vi "SV Read Next Measurement Data.vi"(5 "test signal configuration":refnum<class "SV Signal.lvclass">, 6 "reset start (F)":bool, 7 "reader ID":string="MeasurementData", 8 "error in (no error)":errorcluster, 9 "timeout (1000 ms)":i32=1000, 10 "block length (-1 = all)":i32=-1, 11 "buffer":refnum<data-value>) -> (0 "error out":errorcluster, 1 "end of buffer":bool, 2 "waveforms subset":waveform(dbl)[](array[waveform]), 3 "buffer out":refnum<data-value>, 4 "done":bool)   [LabVIEW 2017]
doc: "Adds buffering to stimulus-response applications. You must manually select the polymorphic instance to use."
uses:
  <vilib>/addons/_NISVFA/_Generation/Signal Generation/SV Signal/SV Signal.lvclass
  <vilib>/addons/_NISVFA/_Shared subVIs/Data Objects/Waveforms (DBL)/Waveforms (N Ch).lvclass
  C:/Program Files (x86)/National Instruments/LabVIEW 2017/vi.lib/addons/_NISVFA/_Shared subVIs/Data Objects/Data/Data.lvclass
  <vilib>/addons/_NISVFA/_Shared subVIs/Data Objects/Data/Data.lvclass/Data.ctl
  <vilib>/addons/_NISVFA/_Shared subVIs/Common/sv_Get NI Property Name String.vi
  <vilib>/addons/_NISVFA/_Generation/Signal Generation/SV Signal/Write Sample Rate.vi
  <vilib>/addons/_NISVFA/_Generation/Signal Generation/SV Signal/Read Sample Rate.vi
  <vilib>/addons/_NISVFA/_Shared subVIs/Data Objects/Data/Data.lvclass
  <vilib>/addons/_NISVFA/_Generation/SoundVib_Generation.lvlib
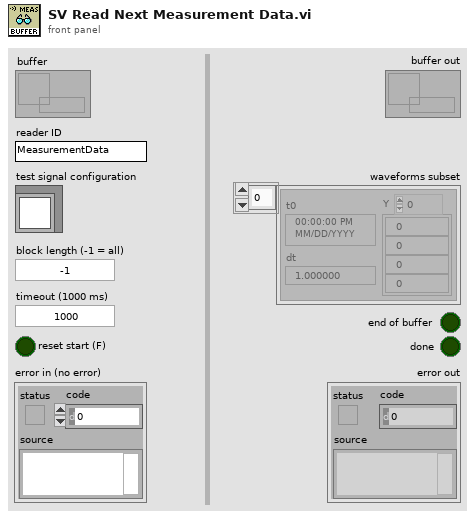
[diagram p1: front panel]
types:
  T1 = typedef "SV Signal.lvclass/sv_System Timing Model.ctl" = i64
  T2 = typedef "SV Signal.lvclass/sv_Generation State.ctl" = enum16{"Idle", "Ramp Up", "Pre-Measurement Settling", "Measurement", "Post-Measurement Settling", "Discrete Sweep Transition", "Ramp Down", "Update"}
  T3 = cluster{"system timing model":T1, "state":cluster{"RESET":bool, "generator timestamp":timestamp, "elapsed seconds":dbl, "elapsed samples":u64, "generation state":T2, "time offset at state":dbl, "samples generated at state":u64, "signal state":variant}, "duration of state":dbl, "samples remaining at state":i32}
  T4 = typedef "SoundVib_Generation.lvlib/sv_Chirp Settings.ctl" = cluster{"amplitude":dbl, "frequency range":cluster{"start (Hz)":dbl, "stop (Hz)":dbl, "frequency spacing":enum16{"Linear", "Logarithmic"}}, "sampling info":cluster{"Fs":dbl, "chirp duration [s]":dbl}, "initial states":cluster{"frequency [Hz]":dbl, "phase [rad]":dbl, "elapsed time [s]":dbl}, "frequency slope":dbl, "maximum harmonic":i32, "prefix len [samples]":cluster{"integer":u32, "fractional":dbl}}
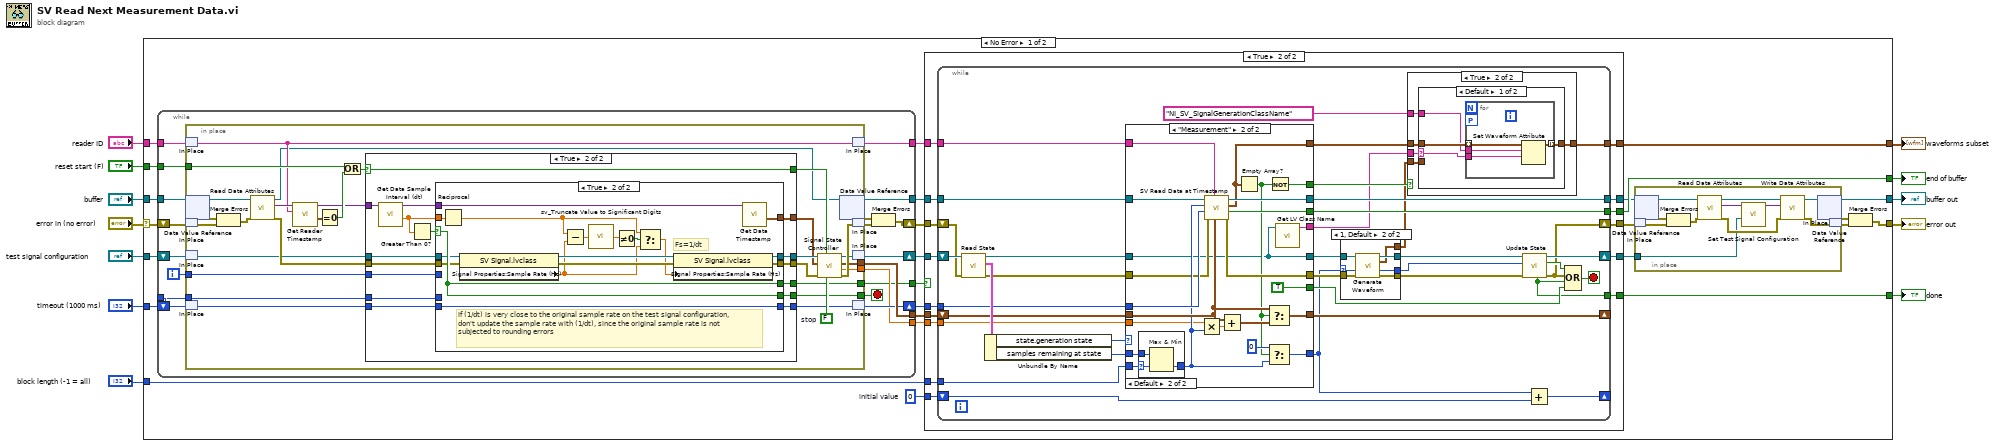
[diagram p0: block diagram]
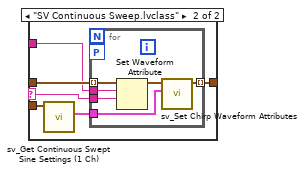
[diagram p5: hidden frame]
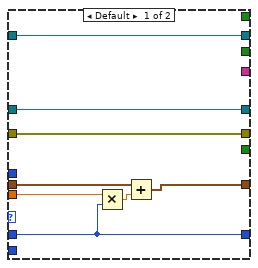
[diagram p6: hidden frame]
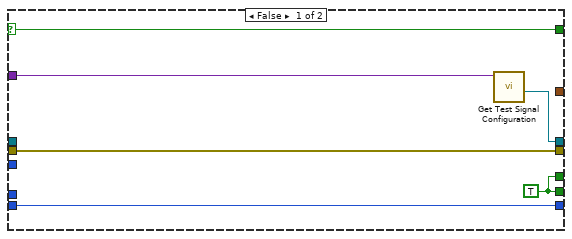
[diagram p8: hidden frame]
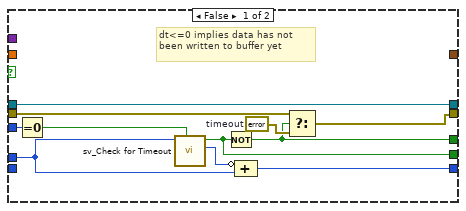
[diagram p9: hidden frame]
diagram:
  n1 = case shown="No Error" "error in (no error)" {
    selector: "error in (no error)" -> [w19 w273]
    tunnel: [w38 w273] -> w12
    tunnel: [w37 _] -> w11
    tunnel: "block length (-1 = all)" -> [w36 _]
    tunnel: "reset start (F)" -> [w35 _]
    tunnel: [w34 _] -> w8
    tunnel: [w33 _] -> w7
    tunnel: [w31 w274] -> w6
    tunnel: "reader ID" -> [w32 _]
    tunnel: "buffer" -> [w29 w274]
    tunnel: "test signal configuration" -> [w18 _]
    tunnel: "timeout (1000 ms)" -> [w15 _]
    frame No Error {
      w30 = 0  # initial value
      n2 = while {
        tunnel: w35 -> [w182]
        tunnel: w32 -> [w181]
        tunnel: w29 -> [w180]
        tunnel: [w178] -> w28
        tunnel: [w177] -> w22
        tunnel: [w175] -> w20
        shift-right: [w176] -> w21
        shift-left: w19 -> [w174]
        shift-right: [w171] -> w17
        shift-left: w18 -> [w172]
        shift-right: [w169] -> w16
        shift-left: w15 -> [w170]
        tunnel: w15 -> [w168]
        tunnel: [w165] -> w14
        tunnel: [w164] -> w13
        i -> [w166]
        stop <- w167 stop-if-true
        n3 = in-place {
          in-place-border: w182 -> [w204]
          in-place-border: [w196] -> w175
          in-place-border: w168 -> [w187]
          in-place-border: [w186] -> w167
          in-place-border: w166 -> [w185]
          in-place-border: [w184] -> w165
          in-place-border: [w183] -> w164
          w195 = FALSE  # stop
          n4 = in-place-match #1(w181) -> (w201:string)
          n5 = in-place-dvr #2(w180) -> (w211:refnum<class "Waveforms (N Ch).lvclass">, w210:errorcluster)
          n6 = in-place-match #3(w174) -> (w193:errorcluster)
          n7 = in-place-match #4(w172) -> (w192:refnum<class "SV Signal.lvclass">)
          n8 = in-place-match #5(w170) -> (w189:i32)
          n9 = Merge Errors(w210, w193) -> (w209:errorcluster)
          n10 = call <vilib>:"Read Data Attributes.vi"("error in (no error)"=w209, "Data in"=w211) -> ("error out"=w208:errorcluster, "data attributes"=w206:variant, "Data out"=w190:refnum<class "Waveforms (N Ch).lvclass">)  [unwired: 7 in]
          n11 = call <vilib>:"Get Reader Timestamp.vi"("ID"=w201, "data attributes"=w206) -> ("timestamp"=w203:timestamp, "data attributes"=w205:variant)  [unwired: 8 in]
          n12 = Equal To 0?(x=w203) -> (x = 0?=w207:bool)
          n13 = Or(x=w204, y=w207) -> (x .or. y?=w202:bool)
          n14 = case shown="True" w202 {
            selector: w202 -> [w214 w228]
            tunnel: w192 -> [_ w232]
            tunnel: w205 -> [w216 w227]
            tunnel: w208 -> [w217 w233]
            tunnel: [w217 w230] -> w198
            tunnel: [w215 w231] -> w200
            tunnel: [_ w229] -> w199
            tunnel: [w214 w228] -> w194
            tunnel: w189 -> [w213 w224]
            tunnel: [w213 w226] -> w188
            tunnel: w187 -> [_ w225]
            tunnel: [w212 w223] -> w186
            tunnel: w185 -> [_ w222]
            tunnel: [w212 w218] -> w183
            frame False {
              w212 = TRUE ("timeout")
              n15 = call <vilib>:"Get Test Signal Configuration.vi"("variant in"=w216) -> ("signal configuration"=w215:refnum<class "SV Signal.lvclass">)  [unwired: 9 in, 1 out]
            }
            frame True {
              n16 = call <vilib>:"Get Data Sample Interval (dt).vi"("variant in"=w227) -> ("dt [s]"=w219:dbl, "variant out"=w221:variant)  [unwired: 9 in]
              n17 = Greater Than 0?(x=w219) -> (x > 0?=w220:bool)
              n18 = case shown="True" w220 {
                selector: w220 -> [_ w255]
                tunnel: w233 -> [w237 w253]
                tunnel: w232 -> [w244 w254]
                tunnel: [w244 w261] -> w231
                tunnel: [w242 w260] -> w230
                tunnel: [_ w259] -> w229
                tunnel: w221 -> [_ w258]
                tunnel: w219 -> [_ w257]
                tunnel: w225 -> [w240 _]
                tunnel: [w239 w255] -> w223
                tunnel: w224 -> [_ w256]
                tunnel: [w238 w256] -> w226
                tunnel: w222 -> [w236 _]
                tunnel: [w234 w255] -> w218
                frame False {
                  w235 = errorcluster {"status"=FALSE, "code"=4990, "source"="samples not available yet"}  # timeout
                  # "dt<=0 implies data has not been written to buffer yet"
                  n19 = Equal To 0?(x=w236) -> (x = 0?=w243:bool)
                  n20 = call <vilib>:"sv_Check for Timeout.vi"("reset"=w243, "timeout [ms]"=w240) -> ("elapsed time [ms]"=w241:i32, "timeout"=w239:bool)  [unwired: 8 in]
                  n21 = Not(x=w239) -> (.not. x?=w234:bool)
                  n22 = Compound Arithmetic op=ADD(invert w241, w240) -> (w238:i32)
                  n23 = Select(t=w237, s=w234, f=w235) -> (s? t:f=w242:errorcluster)
                }
                frame True {
                  # "If (1/dt) is very close to the original sample rate on the test signal configuration, don't update the sample rate with (1/dt), since the original sample rate is not subjected to rounding errors"
                  # "Fs=1/dt"
                  n24 = Reciprocal(x=w257) -> (1/x=w250:dbl)
                  n25 = property class="SV Signal.lvclass"(reference=w254, error in=w253) -> (reference out=w251:refnum<class "SV Signal.lvclass">, error out=w252:errorcluster, "Signal Properties:Sample Rate (Hz)"=w249:dbl)
                  n26 = Subtract(x=w250, y=w249) -> (x-y=w247:dbl)
                  n27 = call <vilib>:"sv_Truncate Value to Significant Digits.vi"("value"=w247) -> ("truncated value"=w246:dbl)  [unwired: 14 in]
                  n28 = Not Equal To 0?(x=w246) -> (x != 0?=w245:bool)
                  n29 = Select(t=w250, s=w245, f=w249) -> (s? t:f=w248:dbl)
                  n30 = property class="SV Signal.lvclass"(reference=w251, error in=w252, "Signal Properties:Sample Rate (Hz)"=w248) -> (reference out=w261:refnum<class "SV Signal.lvclass">, error out=w260:errorcluster)
                  n31 = call <vilib>:"Get Data Timestamp.vi"("variant in"=w258) -> ("timestamp"=w259:timestamp)  [unwired: 9 in, 1 out]
                }
              }
            }
          }
          n32 = call <vilib>:"Signal State Controller.vi"("stop"=w195, "reset"=w194, "error IO"=w198, "current time"=w199, "signal configuration"=w200) -> ("error out"=w197:errorcluster, "waveform dt"=w184:dbl, "waveform t0"=w196:timestamp, "signal configuration"=w191:refnum<class "SV Signal.lvclass">)  [unwired: 3 in]
          n33 = in-place-dvr #2(w190) -> (w178:refnum<data-value>, w179:errorcluster)
          n34 = in-place-match #1(w201) -> (w177:string)
          n35 = in-place-match #3(w197) -> (w173:errorcluster)
          n36 = in-place-match #4(w191) -> (w171:refnum<class "SV Signal.lvclass">)
          n37 = in-place-match #5(w188) -> (w169:i32)
        }
        n38 = Merge Errors(w179, w173) -> (w176:errorcluster)
      }
      n39 = case shown="True" w13 {
        tunnel: [_ w56] -> w37
        tunnel: w36 -> [_ w55]
        tunnel: [_ w54] -> w34
        tunnel: [_ w53] -> w33
        tunnel: w30 -> [_ w52]
        tunnel: w28 -> [w41 w51]
        tunnel: [w41 w50] -> w27
        tunnel: [w39 w49] -> w26
        tunnel: [w40 w48] -> w24
        tunnel: w22 -> [_ w47]
        tunnel: w21 -> [w40 w46]
        tunnel: w20 -> [_ w45]
        tunnel: w17 -> [w39 w44]
        tunnel: w16 -> [_ w43]
        tunnel: w14 -> [_ w42]
        frame False {
        }
        frame True {
          n40 = while {
            shift-right: [w88] -> w49
            shift-left: w44 -> [w91]
            shift-right: [w89] -> _
            shift-left: w52 -> [w92]
            shift-right: [w69] -> w48
            shift-left: w46 -> [w90]
            shift-right: [w78] -> _
            shift-left: w45 -> [w81]
            tunnel: w55 -> [w82]
            tunnel: w51 -> [w70]
            tunnel: [w65] -> w56
            tunnel: w47 -> [w80]
            tunnel: w43 -> [w79]
            tunnel: [w63] -> w50
            tunnel: [w77] -> w54
            tunnel: [w68] -> w53
            tunnel: w42 -> [w67]
            stop <- w83 stop-if-true
            n41 = call <vilib>:"Read State.vi"("error in (no error)"=w90, "signal configuration"=w91) -> ("error out"=w60:errorcluster, "generator state"=w87:T3, "signal configuration"=w61:refnum<class "SV Signal.lvclass">)  [unwired: 7 in]
            n42 = Unbundle By Name(w87) -> ("state.generation state"=w86:T2, "samples remaining at state"=w85:i32)
            n43 = case shown="\"Measurement\"" w86 {
              tunnel: w82 -> [_ w159]
              tunnel: [w134 w145] -> w71
              tunnel: w85 -> [w134 w158]
              tunnel: [_ TRUE] -> w84
              tunnel: w70 -> [w132 w156]
              tunnel: w81 -> [w135 w150]
              tunnel: w60 -> [w130 w141]
              tunnel: [w130 w142] -> w72
              tunnel: [w131 w139] -> w74
              tunnel: [_ w152] -> w66
              tunnel: w80 -> [_ w155]
              tunnel: w79 -> [_ w154]
              tunnel: [w133 w148] -> w78
              tunnel: [w132 w153] -> w63
              tunnel: [_ w144] -> w77
              tunnel: w61 -> [w131 w139]
              tunnel: w67 -> [w129 w143]
              tunnel: [_ w137] -> w64
              tunnel: [_ w138] -> w59
              frame Default {
                n44 = Multiply(x=w129, y=w134) -> (x*y=w136:dbl)
                n45 = Add(x=w135, y=w136) -> (x+y=w133:timestamp)
              }
              frame "Measurement" {
                n46 = case shown="Default" w159 {
                  selector: w159 -> [_ w161]
                  tunnel: w158 -> [w160 w163]
                  tunnel: [w160 w162] -> w146
                  frame ..-1 {
                  }
                  frame Default {
                    n47 = Max & Min(x=w163, y=w161) -> (min(x,y)=w162:i32)  [unwired: 1 out]
                  }
                }
                n48 = Multiply(x=w143, y=w146) -> (x*y=w151:dbl)
                n49 = call <vilib>:"SV Read Data at Timestamp.vi"("timestamp (first available)"=w150, "reader ID"=w155, "error in (no error)"=w141, "timeout (0 ms)"=w154, "block length (-1 = all)"=w146, "buffer"=w156) -> ("error out"=w142:errorcluster, "end of buffer"=w144:bool, "waveforms subset"=w152:waveform(dbl)[], "buffer out"=w153:refnum<data-value>)  [unwired: 2 in]
                n50 = Add(x=w150, y=w151) -> (x+y=w149:timestamp)
                n51 = Empty Array?(array=w152) -> (empty?=w140:bool)
                n52 = Select(t=w150, s=w140, f=w149) -> (s? t:f=w148:timestamp)
                n53 = Select(t=0, s=w140, f=w146) -> (s? t:f=w145:i32)
                n54 = Not(x=w140) -> (.not. x?=w137:bool)
                n55 = call <vilib>:"Get LV Class Name.vi"("object"=w139) -> ("class name"=w138:string)  [unwired: 9 in, 1 out]
              }
            }
            n56 = case shown="1, Default" w71 {
              selector: w71 -> [w93 w98]
              tunnel: [w95 w102] -> w75
              tunnel: w74 -> [w95 w101]
              tunnel: [w94 w100] -> w73
              tunnel: w72 -> [w94 w99]
              tunnel: [_ w97] -> w62
              tunnel: [w93 w96] -> w57
              frame ..0 {
              }
              frame 1, Default {
                n57 = call-dynamic "Generate Waveform.vi"("signal configuration and state in"=w101, "samples"=w98, "error in (no error)"=w99) -> ("signal configuration and state out"=w102:refnum<class "SV Signal.lvclass">, "output waveform"=w97:waveform(dbl), "samples"=w96:i32, "error out"=w100:errorcluster)  [unwired: 9 in]
              }
            }
            n58 = case shown="True" w64 {
              tunnel: w66 -> [w103 w108]
              tunnel: [w103 w107] -> w65
              tunnel: w62 -> [_ w106]
              tunnel: w59 -> [_ w105]
              tunnel: "NI_SV_SignalGenerationClassName" -> [_ w104]
              frame False {
              }
              frame True {
                n59 = case shown="Default" w105 {
                  selector: w105 -> [w110 w118]
                  tunnel: w108 -> [w112 w122]
                  tunnel: [w111 w121] -> w107
                  tunnel: w106 -> [_ w120]
                  tunnel: w104 -> [w109 w117]
                  frame Default {
                    n60 = for {
                      tunnel: [w116] -> w111 mode=indexing
                      workers-P: _ -> [_]
                      tunnel: w110 -> [w115]
                      tunnel: w109 -> [w114]
                      tunnel: w112 -> [w113] mode=indexing
                      n61 = Set Waveform Attribute(5:w115, 6:w114, 7:w113) -> (3:w116:waveform(dbl))  [unwired: 1 in, 2 out]
                    }
                  }
                  frame "SV Continuous Sweep.lvclass" {
                    n62 = call <vilib>:"sv_Get Continuous Swept Sine Settings (1 Ch).vi"("waveform"=w120) -> ("chirp settings out"=w119:T4)  [unwired: 8 in, 2 out]
                    n63 = for {
                      tunnel: w122 -> [w125] mode=indexing
                      tunnel: [w123] -> w121 mode=indexing
                      tunnel: w119 -> [w128]
                      workers-P: _ -> [_]
                      tunnel: w118 -> [w127]
                      tunnel: w117 -> [w126]
                      n64 = Set Waveform Attribute(5:w127, 6:w126, 7:w125) -> (3:w124:waveform(dbl))  [unwired: 1 in, 2 out]
                      n65 = call <vilib>:"sv_Set Chirp Waveform Attributes.vi"("chirp settings"=w128, "chirp signal"=w124) -> ("chirp signal out"=w123:waveform(dbl))  [unwired: 8 in, 1 out]
                    }
                  }
                }
              }
            }
            n66 = call-dynamic "Update State.vi"("error in (no error)"=w73, "samples generated"=w57, "signal configuration"=w75) -> ("error out"=w69:errorcluster, "generation done"=w76:bool, "signal configuration"=w88:refnum<class "SV Signal.lvclass">, "measurement done"=w68:bool)  [unwired: 4 in, 1 out]
            n67 = Add(x=w71, y=w92) -> (x+y=w89:i32)
            n68 = Compound Arithmetic op=OR(w76, w69, w68, w84) -> (w83:bool)
          }
        }
      }
      n69 = in-place {
        in-place-border: w26 -> [w266]
        n70 = in-place-dvr #6(w27) -> (w272:refnum<class "Waveforms (N Ch).lvclass">, w265:errorcluster)
        n71 = in-place-match #7(w24) -> (w263:errorcluster)
        n72 = Merge Errors(w265, w263) -> (w264:errorcluster)
        n73 = call <vilib>:"Read Data Attributes.vi"("error in (no error)"=w264, "Data in"=w272) -> ("error out"=w267:errorcluster, "data attributes"=w271:variant, "Data out"=w269:refnum<class "Waveforms (N Ch).lvclass">)  [unwired: 7 in]
        n74 = call <vilib>:"Set Test Signal Configuration.vi"("signal configuration"=w266, "variant in"=w271) -> ("variant out"=w270:variant)  [unwired: 9 in]
        n75 = call <vilib>:"Write Data Attributes.vi"("error in (no error)"=w267, "data attributes"=w270, "Data in"=w269) -> ("error out"=w262:errorcluster, "Data out"=w268:refnum<class "Waveforms (N Ch).lvclass">)  [unwired: 7 in]
        n76 = in-place-dvr #6(w268) -> (w31:refnum<data-value>, w25:errorcluster)
        n77 = in-place-match #7(w262) -> (w23:errorcluster)
      }
      n78 = Merge Errors(w25, w23) -> (w38:errorcluster)
    }
    frame Error {
    }
  }
  "error out" <- w12
  "waveforms subset" <- w11
  "end of buffer" <- w8
  "done" <- w7
  "buffer out" <- w6
